vi "Add Pulse Recorder.vi"(6 "Reset":bool, 8 "error in (no error)":errorcluster, 9 "Auto launch":bool=TRUE, 10 "Module type":T1, 11 "LabActor in":refnum<class "LabActor.lvclass">) -> (0 "error out":errorcluster, 3 "LabActor out":refnum<class "LabActor.lvclass">)   [LabVIEW 2018, in "LabActor.lvclass"]
uses:
  LabActor.lvclass
  C:/github/LabActor/Controllers/Application Controller/Application Controller.lvclass
  Controllers/Application Controller/Module Types.ctl
  LabActor.lvclass/LabActor.ctl
  Controllers/Application Controller/Application Controller.lvclass/Application Controller.ctl
  Controllers/Application Controller/Read Monitor ref.vi
  NHMFL_Core/Libraries/Queued Listbox/Queued Listbox.xctl
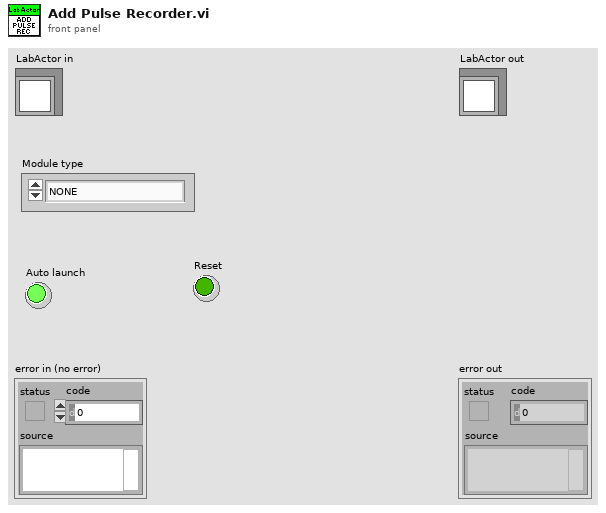
[diagram p1: front panel]
types:
  T1 = typedef "Module Types.ctl" = enum16{"NONE", "NI-DAQmx", "NI-Scope", "Red Pitaya Digitizer", "GaGe", "VISA Device", "Red Pitaya Lockin", "Monitor Controller", "Pulse Controller", "Integrate Pulse", "Lockin Processor", "File converter", "NHMFL Synthesizer", "Micron Hyperion", "Spectrum Recorder", "Resonance Detector", "TCP Communications", "Format Resonances", "Ruby Spectra", "PID Controller", "Quantum Design"}
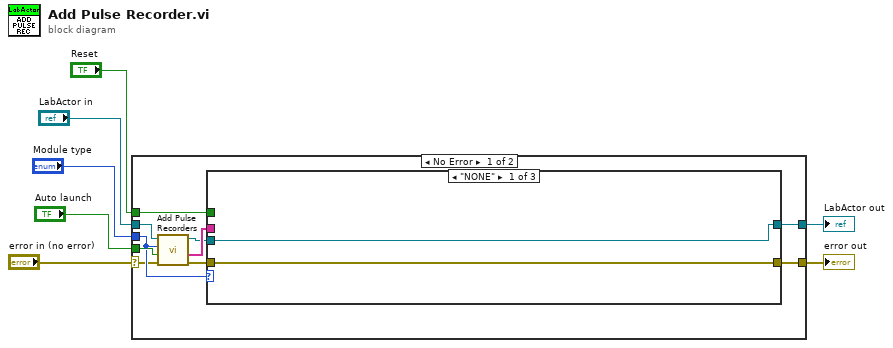
[diagram p0: block diagram]
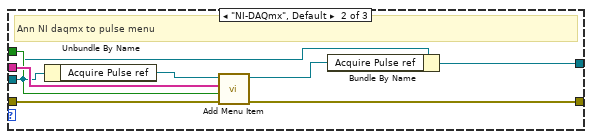
[diagram p2: hidden frame]
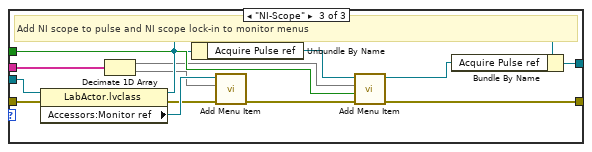
[diagram p3: hidden frame]
diagram:
  n1 = case shown="No Error" "error in (no error)" {
    selector: "error in (no error)" -> [w11 w43]
    tunnel: [w10 w43] -> w6
    tunnel: [w12 w42] -> w4
    tunnel: "LabActor in" -> [w8 w42]
    tunnel: "Module type" -> [w16 _]
    tunnel: "Auto launch" -> [w17 _]
    tunnel: "Reset" -> [w14 _]
    frame No Error {
      n2 = call-dynamic "Add Pulse Recorders.vi"("error in (no error)"=w11, "Auto launch"=w17, "Module type"=w16, "LabActor in"=w8) -> ("error out"=w13:errorcluster, "Actor names out"=w15:string[], "LabActor out"=w9:refnum<class "LabActor.lvclass">)  [unwired: 3 in, 2 out]
      n3 = case shown="\"NONE\"" w16 {
        tunnel: w9 -> [w18 w23 w35]
        tunnel: w15 -> [_ w26 w40]
        tunnel: w14 -> [_ w25 w39]
        tunnel: w13 -> [w19 w24 w38]
        tunnel: [w18 w21 w36] -> w12
        tunnel: [w19 w20 w30] -> w10
        frame "NONE" {
        }
        frame "NI-DAQmx", Default {
          # "Ann NI daqmx to pulse menu"
          n4 = Unbundle By Name(w23) -> ("Acquire Pulse ref"=w27:refnum<vi>)
          n5 = call "Add Menu Item.vi"("error in (no error)"=w24, "Reset"=w25, "Item Names"=w26, "Queed Listbox ref"=w27) -> ("error out"=w20:errorcluster, "Queed Listbox ref out"=w22:refnum<vi>)  [unwired: 5 in, 1 out]
          n6 = Bundle By Name(cluster=w23, "Acquire Pulse ref"=w22) -> (w21:refnum<class "LabActor.lvclass">)
        }
        frame "NI-Scope" {
          # "Add NI scope to pulse and NI scope lock-in to monitor menus"
          n7 = property class="LabActor.lvclass"(reference=w35, error in=w38) -> (reference out=w34:refnum<class "LabActor.lvclass">, error out=w28:errorcluster, "Accessors:Monitor ref"=w33:refnum<vi>)
          n8 = Decimate 1D Array(w40) -> (w32:string[], w31:string[])
          n9 = Unbundle By Name(w34) -> ("Acquire Pulse ref"=w41:refnum<vi>)
          n10 = call "Add Menu Item.vi"("error in (no error)"=w28, "Item Names"=w31, "Queed Listbox ref"=w33) -> ("error out"=w29:errorcluster)  [unwired: 6 in, 2 out]
          n11 = call "Add Menu Item.vi"("error in (no error)"=w29, "Reset"=w39, "Item Names"=w32, "Queed Listbox ref"=w41) -> ("error out"=w30:errorcluster, "Queed Listbox ref out"=w37:refnum<vi>)  [unwired: 5 in, 1 out]
          n12 = Bundle By Name(cluster=w34, "Acquire Pulse ref"=w37) -> (w36:refnum<class "LabActor.lvclass">)
        }
      }
    }
    frame Error {
    }
  }
  "error out" <- w6
  "LabActor out" <- w4
